vi "CMD.vi"(4 "error in (no error)":errorcluster, 5 "PMU ID":u16, 7 "command":T1=enum."Turn on Transmission of Data Frame" format="%04b") -> (0 "error out":errorcluster, 3 "CMD":string)   [LabVIEW 2013]
uses:
  CTRLs/PMU_CMDs.ctl
  CTRLs/PMU_CFG Class.ctl
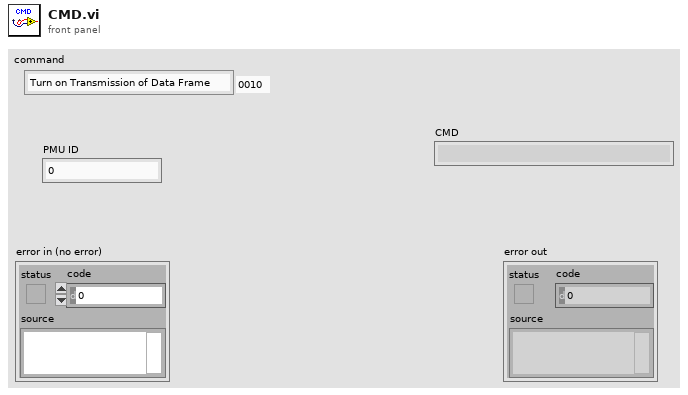
[diagram p1: front panel]
types:
  T1 = typedef "PMU_CMDs.ctl" = enum16{"dummy", "Turn off Transmission of Data Frame", "Turn on Transmission of Data Frame", "Send Header Frame", "Send CFG-1 Frame", "Send CFG-2 Frame", "Extended Frame"}
  T2 = typedef "PMU_CFG Class.ctl" = cluster{"station name":string, "PMU ID":u16, "time base":u32, "nominal frequency":enum16{"50 Hz", "60 Hz"}, "reporting rate":i16, "phasor number":u16, "analog number":u16, "digital number":u16, "channel names":string[], "phasor units":u32[], "analog units":u32[], "digital units":u32[], "data format":u16, "number of PMUs":u16}
  T3 = typedef "LVDateTimeRec.ctl" = cluster{"fractional second":dbl, "second":i32, "minute":i32, "hour":i32, "day of month":i32, "month":i32, "year":i32, "day of week":i32, "day of year":i32, "DST":i32}
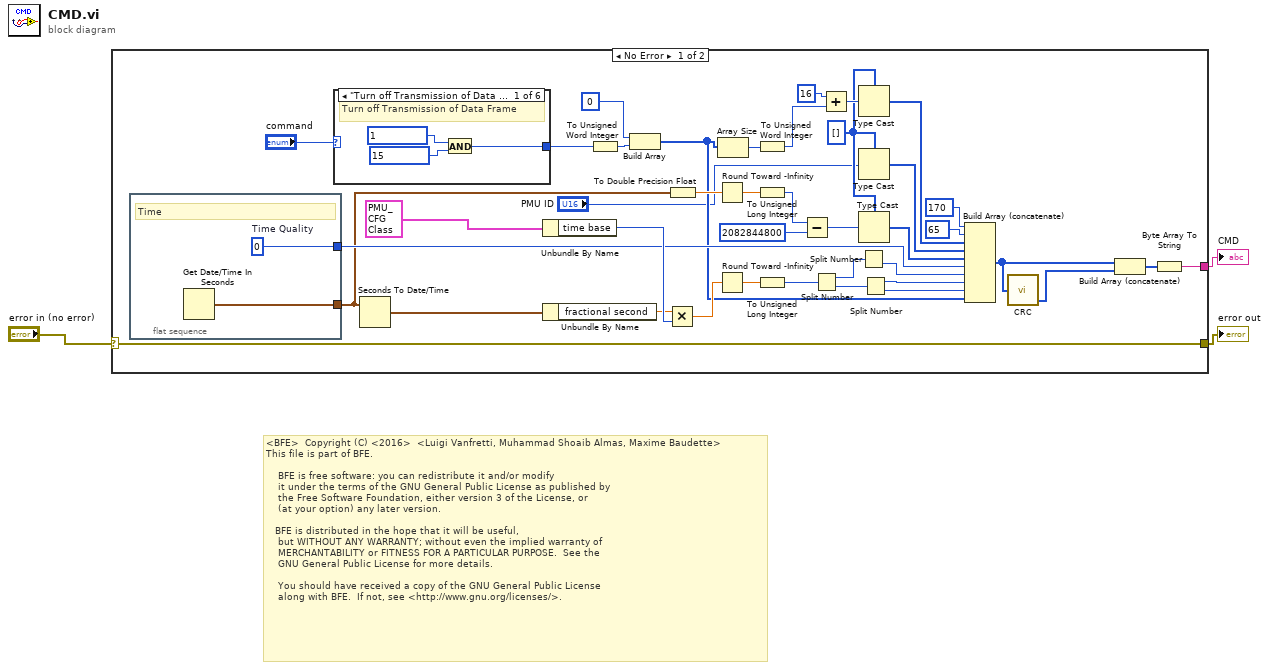
[diagram p0: block diagram]
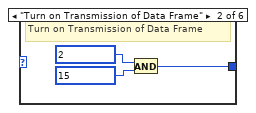
[diagram p2: hidden frame]
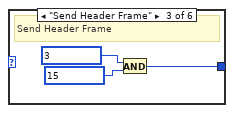
[diagram p3: hidden frame]
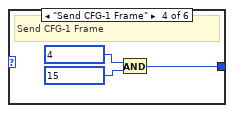
[diagram p4: hidden frame]
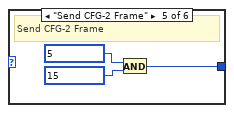
[diagram p5: hidden frame]
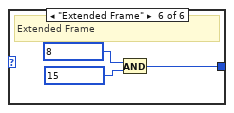
[diagram p6: hidden frame]
diagram:
  # "<BFE>  Copyright (C) <2016>  <Luigi Vanfretti, Muhammad Shoaib Almas, Maxime Baudette> \nThis file is part of BFE.\n\n    BFE is free software: you can redistribute it and/or modify\n    it under the terms of the GNU General Public License as published by\n    the Free Software Foundation, either version 3 of the License, or\n    (at your option) any later version.\n\n   BFE is distributed in the hope that it will be useful,\n    but WITHOUT ANY WARRANTY; without even the implied warranty of\n    MERCHANTABILITY or FITNESS FOR A PARTICULAR PURPOSE.  See the\n    GNU General Public License for more details.\n\n    You should have received a copy of the GNU General Public License\n    along with BFE.  If not, see <http://www.gnu.org/licenses/>."
  n1 = case shown="No Error" "error in (no error)" {
    selector: "error in (no error)" -> [w15 w64]
    tunnel: [w43 _] -> w3
    tunnel: [w15 w64] -> w2
    frame No Error {
      w28 = u8[] [] ("appended array")
      n2 = flat-sequence {
        tunnel: [w63] -> w18
        tunnel: [w62] -> w17
        frame #0 {
          w63 = u8 0  # Time Quality
          # "Time"
          n3 = Get Date/Time In Seconds() -> (seconds since 1Jan1904=w62:timestamp)
        }
      }
      n4 = case shown="\"Turn off Transmission of Data Frame\", Default" "command" {
        tunnel: [w45 w48 w51 w54 w57 w60] -> w12
        frame "Turn off Transmission of Data Frame", Default {
          # "Turn off Transmission of Data Frame"
          n5 = And(x=u16 1 ("y"), y=u16 15) -> (x .and. y?=w45:u16)
        }
        frame "Turn on Transmission of Data Frame" {
          # "Turn on Transmission of Data Frame"
          n6 = And(x=u16 2 ("y"), y=u16 15) -> (x .and. y?=w48:u16)
        }
        frame "Send Header Frame" {
          # "Send Header Frame"
          n7 = And(x=u16 3 ("y"), y=u16 15) -> (x .and. y?=w51:u16)
        }
        frame "Send CFG-1 Frame" {
          # "Send CFG-1 Frame"
          n8 = And(x=u16 4 ("y"), y=u16 15) -> (x .and. y?=w54:u16)
        }
        frame "Send CFG-2 Frame" {
          # "Send CFG-2 Frame"
          n9 = And(x=u16 5 ("y"), y=u16 15) -> (x .and. y?=w57:u16)
        }
        frame "Extended Frame" {
          # "Extended Frame"
          n10 = And(x=u16 8 ("y"), y=u16 15) -> (x .and. y?=w60:u16)
        }
      }
      n11 = Seconds To Date/Time(time stamp (now)=w17) -> (date time rec=w16:T3)  [unwired: 1 in]
      n12 = Unbundle By Name(T2 {"station name"="", "PMU ID"=1022, "time base"=10000000, "nominal frequency"=enum."60 Hz", "reporting rate"=60, "phasor number"=0, "analog number"=0, "digital number"=0, "channel names"=[], "phasor units"=[], "analog units"=[], "digital units"=[], "data format"=15, "number of PMUs"=1} ("CFG class")) -> ("time base"=w25:u32)
      n13 = Unbundle By Name(w16) -> ("fractional second"=w14:dbl)
      n14 = To Unsigned Word Integer(number=w12) -> (unsigned 16bit integer=w11:u16)
      n15 = Build Array(u16 0 ("element"), w11) -> (w7:u16[])
      n16 = Multiply(x=w14, y=w25) -> (x*y=w21:dbl)
      n17 = To Double Precision Float(number=w17) -> (double precision float=w23:dbl)
      n18 = Round Toward -Infinity(1:w23) -> (0:w22:dbl)
      n19 = Round Toward -Infinity(1:w21) -> (0:w20:dbl)
      n20 = Array Size(array=w7) -> (size(s)=w41:i32)
      n21 = To Unsigned Word Integer(number=w41) -> (unsigned 16bit integer=w39:u16)
      n22 = To Unsigned Long Integer(number=w22) -> (unsigned 32bit integer=w26:u32)
      n23 = To Unsigned Long Integer(number=w20) -> (unsigned 32bit integer=w27:u32)
      n24 = Subtract(x=w26, y=u32 2082844800 ("unsigned 32bit integer")) -> (x-y=w30:u32)
      n25 = Split Number(x=w27) -> (hi(x)=w36:u16, lo(x)=w37:u16)
      n26 = Add(x=u16 16 ("y"), y=w39) -> (x+y=w32:u16)
      n27 = Type Cast(type=w28, x=w32) -> (*(type *) &x=w31:u8[])
      n28 = Type Cast(type=w28, x="PMU ID") -> (*(type *) &x=w8:u8[])
      n29 = Type Cast(type=w28, x=w30) -> (*(type *) &x=w29:u8[])
      n30 = Split Number(x=w36) -> (lo(x)=w35:u8)  [unwired: 1 out]
      n31 = Split Number(x=w37) -> (hi(x)=w34:u8, lo(x)=w33:u8)
      n32 = Build Array (concatenate)(u8 170 ("element"), u8 65 ("element"), w31, w8, w29, w18, w35, w34, w33, w7) -> (w19:u16[])
      n33 = call "CRC.vi"("byte array"=w19) -> ("CRCbytes"=w10:u8[])  [unwired: 1 out]
      n34 = Build Array (concatenate)(w19, w10) -> (w9:u16[])
      n35 = Byte Array To String(unsigned byte array=w9) -> (string=w43:string)
    }
    frame Error {
    }
  }
  "CMD" <- w3
  "error out" <- w2
